vi "Init Events.vi"(8 "error in (no error)":errorcluster, 11 "TSEngine in":refnum<class "Engine.lvclass">) -> (0 "error out":errorcluster, 3 "TSEngine out":refnum<class "Engine.lvclass">, 4 "Event Reg":refnum<event-registration>, 6 "Events":T1)   [LabVIEW 2019, in "HTS.lvlib" / "Engine.lvclass"]
uses:
  Engine.lvclass
  Variable Container Type.ctl
  Create VC Event Data.ctl
  Events.ctl
  VariableContainer/VariableContainer.lvclass
  VariableContainer/Typedefs/Session Handle.ctl
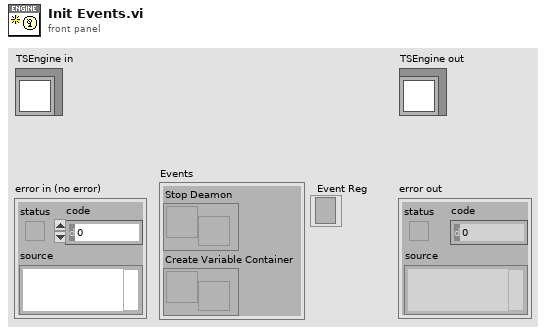
[diagram p1: front panel]
types:
  T1 = typedef "HTS.lvlib/Engine.lvclass/Events.ctl" = cluster{"Stop Deamon":refnum<user-event>, "Create Variable Container":refnum<user-event>}
  T2 = typedef "HTS.lvlib/Engine.lvclass/Create VC Event Data.ctl" = cluster{"Type":T3, "Notifier":refnum<notifier>}
  T3 = typedef "HTS.lvlib/Engine.lvclass/Variable Container Type.ctl" = enum16{"StationGlobals", "TemporaryGlobals", "NewPropertyObject"}
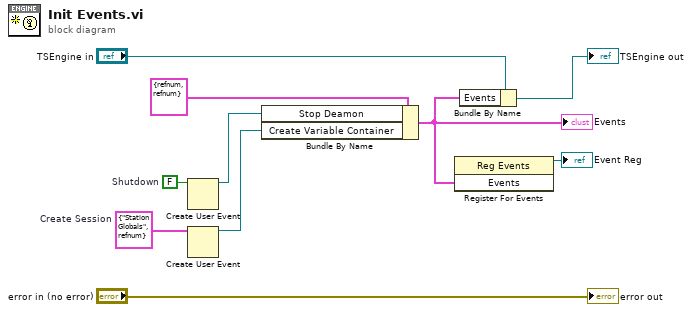
[diagram p0: block diagram]
diagram:
  w6 = T2 {"Type"=enum."StationGlobals", "Notifier"=refnum}  # Create Session
  w9 = FALSE  # Shutdown
  n1 = Create User Event(user event datatype=w9) -> (user event=w4:refnum<user-event>)  [unwired: 1 in, 1 out]
  n2 = Create User Event(user event datatype=w6) -> (user event=w3:refnum<user-event>)  [unwired: 1 in, 1 out]
  n3 = Bundle By Name(cluster=T1 {"Stop Deamon"=refnum, "Create Variable Container"=refnum} ("Events"), "Stop Deamon"=w4, "Create Variable Container"=w3) -> (w2:T1)
  "Events" <- w2
  n4 = register-events(w2) -> (reference out=→"Event Reg":refnum<event-registration>)  [unwired: 2 in, 1 out]
  n5 = Bundle By Name(cluster="TSEngine in", "Events"=w2) -> (→"TSEngine out":refnum<class "Engine.lvclass">)
  "error out" <- "error in (no error)"
